vi "loadHTSocketContactNew.vi"(11 "file (use dialog)":path=path "C:/temp/ht/Socket/MSD6A638JSMG-8-Y8_A151200729_EQC_151220030900.txt") -> ()   [LabVIEW 2012]
uses:
  <vilib>/addons/database/Connection.llb/DB Tools Open Connec (Path).vi
  <vilib>/addons/database/Connection.llb/Conn Execute.vi
  <vilib>/addons/database/Recordset.llb/Rec Fetch Integer Data (R).vi
  <vilib>/addons/database/Recordset.llb/Rec Destroy - Connection.vi
  <vilib>/addons/database/NI_Database_API.lvlib
panel:
  out "array":string[][](array[string])
  out "concatenated string":string
  out "error out":errorcluster
  out "name":string
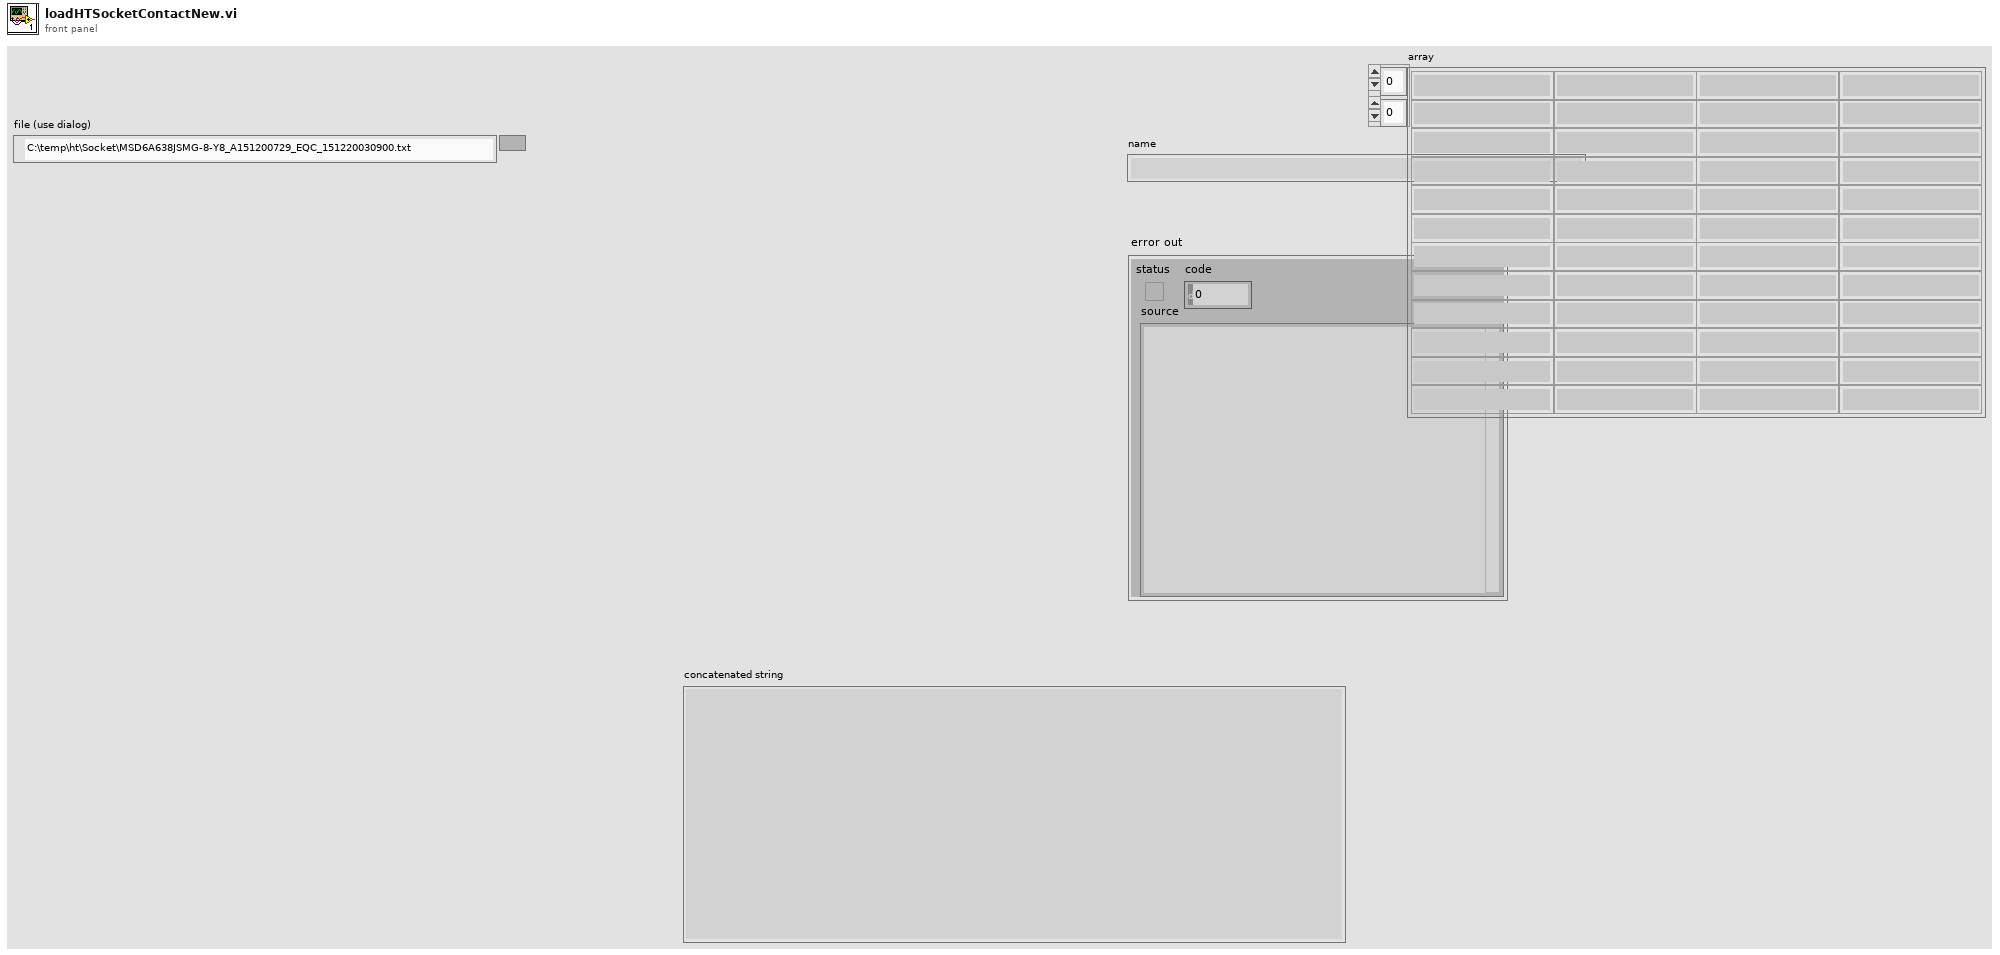
[diagram p1: front panel]
types:
  T1 = typedef "NI_Database_API.lvlib/Conn ObjectReference.ctl" = refnum<k1>
  T2 = typedef "NI_Database_API.lvlib/Rec ObjectReference.ctl" = refnum<k1>
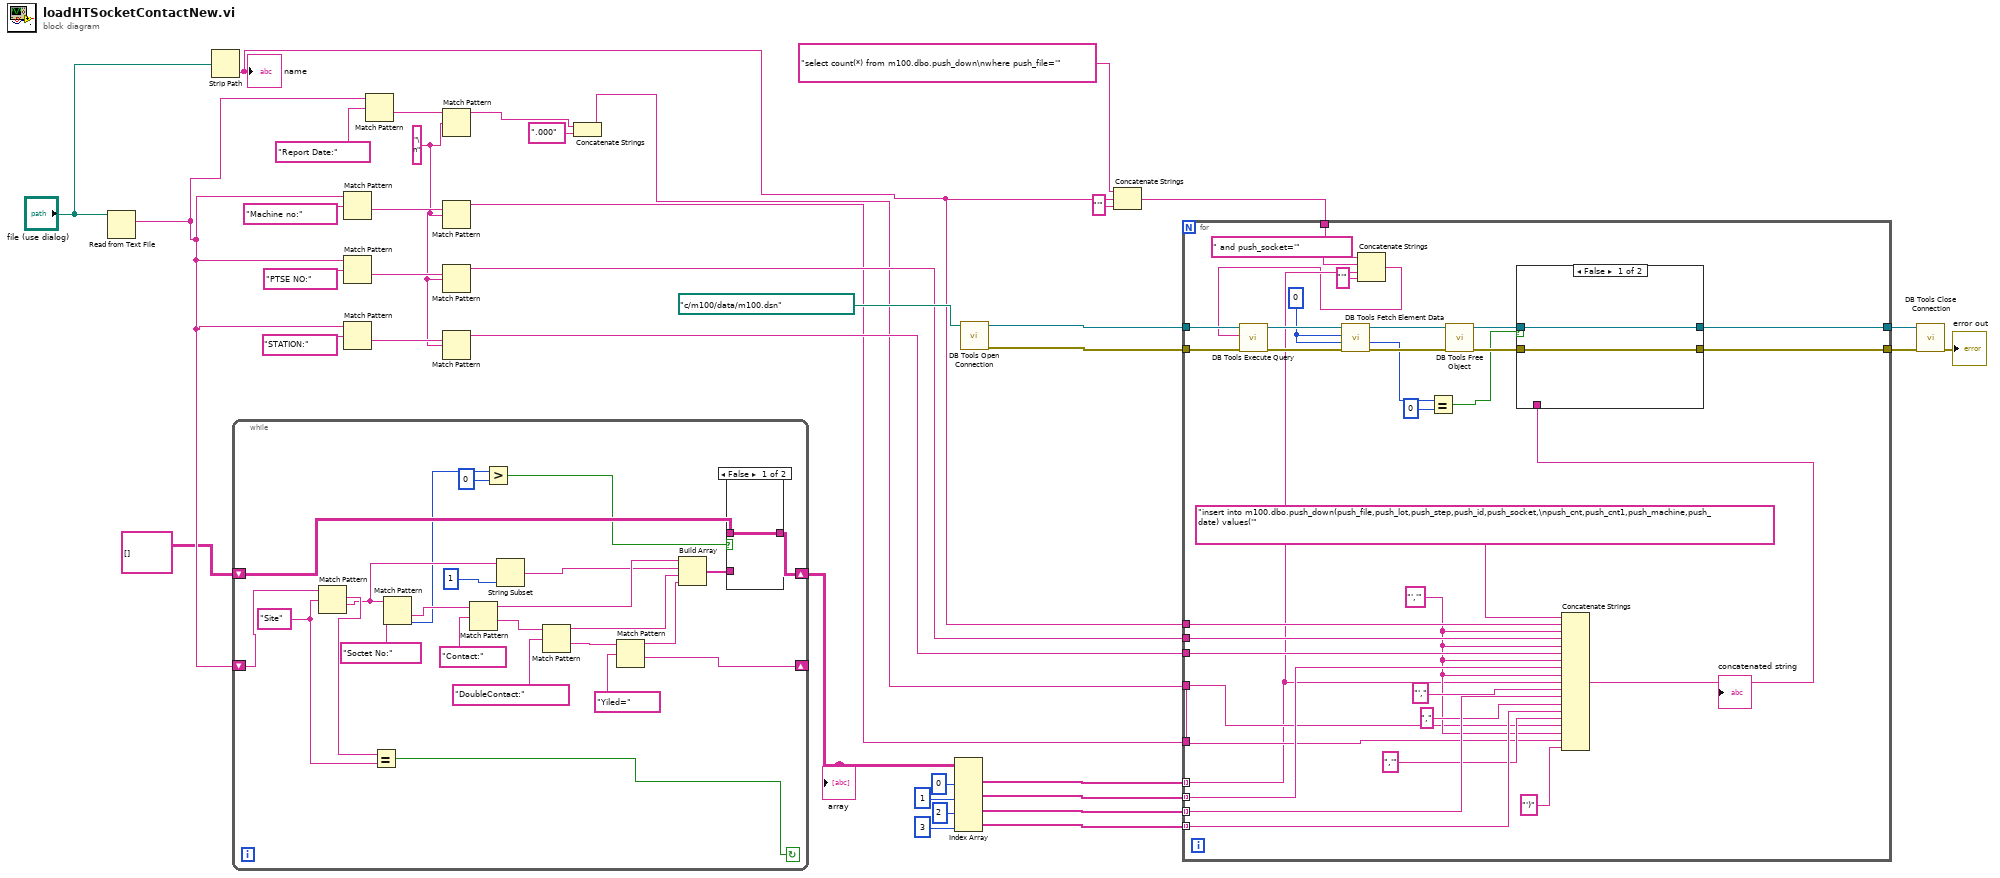
[diagram p0: block diagram]
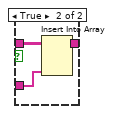
[diagram p2: hidden frame]
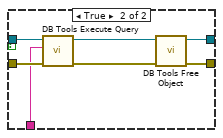
[diagram p3: hidden frame]
diagram:
  w26 = "\n" ("regular expression")
  n1 = Read from Text File(file (use dialog)="file (use dialog)") -> (text=w3:string)  [unwired: 3 in, 3 out]
  n2 = Strip Path(path="file (use dialog)") -> (name=w16:string)  [unwired: 1 out]
  "name" <- w16
  n3 = while {
    shift-right: [w50] -> _
    shift-left: w3 -> [w49]
    shift-right: [w48] -> w1
    shift-left: string[][] [] ("array") -> [w47]
    stop <- w44 continue-if-true
    w45 = "Site" ("regular expression")
    n4 = Match Pattern(string=w49, regular expression=w45) -> (match substring=w46:string, after substring=w41:string)  [unwired: 1 in, 2 out]
    n5 = Equal?(x=w46, y=w45) -> (x = y?=w44:bool)
    n6 = Match Pattern(string=w41, regular expression="Soctet No:") -> (after substring=w43:string, offset past match=w40:i32)  [unwired: 1 in, 2 out]
    n7 = Match Pattern(string=w43, regular expression="Contact:") -> (before substring=w60:string, after substring=w58:string)  [unwired: 1 in, 2 out]
    n8 = Greater?(x=w40, y=0) -> (0:w38:bool)
    n9 = String Subset(string=w41, length (rest)=1 ("length (rest)")) -> (substring=w51:string)  [unwired: 1 in]
    n10 = Match Pattern(string=w58, regular expression="DoubleContact:") -> (before substring=w54:string, after substring=w56:string)  [unwired: 1 in, 2 out]
    n11 = Match Pattern(string=w56, regular expression="Yiled=") -> (before substring=w53:string, after substring=w50:string)  [unwired: 1 in, 2 out]
    n12 = Build Array(w60, w51, w54, w53) -> (w59:string[])
    n13 = case shown="False" w38 {
      tunnel: w59 -> [_ w65]
      tunnel: [w62 w64] -> w48
      tunnel: w47 -> [w62 w63]
      frame False {
      }
      frame True {
        n14 = Insert Into Array(array=w63, new element=w65) -> (w64:string[][])  [unwired: 2 in]
      }
    }
  }
  "array" <- w1
  n15 = Match Pattern(string=w3, regular expression="Machine no:") -> (after substring=w36:string)  [unwired: 1 in, 3 out]
  n16 = Match Pattern(string=w3, regular expression="PTSE NO:") -> (after substring=w29:string)  [unwired: 1 in, 3 out]
  n17 = Match Pattern(string=w3, regular expression="STATION:") -> (after substring=w27:string)  [unwired: 1 in, 3 out]
  n18 = Match Pattern(string=w3, regular expression="Report Date:") -> (after substring=w31:string)  [unwired: 1 in, 3 out]
  n19 = Match Pattern(string=w31, regular expression=w26) -> (before substring=w7:string)  [unwired: 1 in, 3 out]
  n20 = Match Pattern(string=w36, regular expression=w26) -> (before substring=w4:string)  [unwired: 1 in, 3 out]
  n21 = Match Pattern(string=w29, regular expression=w26) -> (before substring=w15:string)  [unwired: 1 in, 3 out]
  n22 = Match Pattern(string=w27, regular expression=w26) -> (before substring=w14:string)  [unwired: 1 in, 3 out]
  n23 = Concatenate Strings(w7, ".000" ("string")) -> (w5:string)
  n24 = Index Array(array=w1, index (col) #1=0 ("disabled index (col)"), index (col) #2=1 ("index (col)"), index (col) #3=2 ("index (col)"), index (col) #4=3 ("index (col)")) -> (element #1=w10:string[], element #2=w11:string[], element #3=w9:string[], element #4=w8:string[])  [unwired: 4 in]
  n25 = call-poly <vilib>:"DB Tools Open Connection.vi"("connection information"=path "c:/m100/data/m100.dsn") -> ("error out"=w23:errorcluster, "connection reference"=w25:T1)  [unwired: 7 in]
  n26 = Concatenate Strings("select count(*) from m100.dbo.push_down\nwhere push_file='", w16, "'" ("string")) -> (w17:string)
  n27 = for {
    tunnel: w25 -> [w99]
    tunnel: [w95] -> w24
    tunnel: w23 -> [w94]
    tunnel: [w90] -> w22
    tunnel: w17 -> [w70]
    tunnel: w16 -> [w84]
    tunnel: w15 -> [w83]
    tunnel: w14 -> [w82]
    tunnel: w11 -> [w81] mode=indexing
    tunnel: w10 -> [w68] mode=indexing
    tunnel: w9 -> [w79] mode=indexing
    tunnel: w8 -> [w77] mode=indexing
    tunnel: w5 -> [w73]
    tunnel: w4 -> [w71]
    w72 = "','" ("string")
    w89 = 0
    n28 = Concatenate Strings(w70, " and push_socket='" ("string"), w68, "'" ("string")) -> (w66:string)
    n29 = call-poly <vilib>:"DB Tools Execute Query.vi"("error in (no error)"=w94, "SQL query"=w66, "connection reference"=w99) -> ("error out"=w93:errorcluster, "recordset reference"=w98:T2)  [unwired: 5 in]
    n30 = call-poly <vilib>:"DB Tools Fetch Element Data.vi"("error in (no error)"=w93, "type"=w89, "column index"=w89, "recordset reference"=w98) -> ("error out"=w92:errorcluster, "data"=w88:i32, "recordset reference out"=w97:T2)  [unwired: 3 in]
    n31 = Equal?(x=w88, y=0) -> (x = y?=w86:bool)
    n32 = call-poly <vilib>:"DB Tools Free Object.vi"("error in (no error)"=w92, "recordset reference"=w97) -> ("error out"=w91:errorcluster, "connection reference"=w96:T1)  [unwired: 8 in]
    n33 = Concatenate Strings("insert into m100.dbo.push_down(push_file,push_lot,push_step,push_id,push_socket,\npush_cnt,push_cnt1,push_machine,push_date) values('", w84, w72, w83, w72, w82, w72, w81, w72, w68, "'," ("string"), w79, "," ("string"), w77, ",'" ("string"), w71, w72, w73, "')" ("string")) -> (w75:string)
    "concatenated string" <- w75
    n34 = case shown="False" w86 {
      tunnel: w96 -> [w101 w108]
      tunnel: [w101 w106] -> w95
      tunnel: w91 -> [w100 w105]
      tunnel: [w100 w103] -> w90
      tunnel: w75 -> [_ w102]
      frame False {
      }
      frame True {
        n35 = call-poly <vilib>:"DB Tools Execute Query.vi"("error in (no error)"=w105, "SQL query"=w102, "connection reference"=w108) -> ("error out"=w104:errorcluster, "recordset reference"=w107:T2)  [unwired: 5 in]
        n36 = call-poly <vilib>:"DB Tools Free Object.vi"("error in (no error)"=w104, "recordset reference"=w107) -> ("error out"=w103:errorcluster, "connection reference"=w106:T1)  [unwired: 8 in]
      }
    }
  }
  n37 = call <vilib>:"DB Tools Close Connection.vi"("error in (no error)"=w22, "connection reference"=w24) -> ("error out"=→"error out":errorcluster)  [unwired: 5 in]
